vi "TruncU64.vi"(5 "Decimal places":i8, 6 "Number":u64) -> (2 "Truncated number":u64)   [LabVIEW 2017, in "GPNumeric.lvlib"]
doc: "Truncates <B>Number</B> to a number of <B>Decimal places</B>.\n\nSet <B>Decimal places</B> to a negative number to truncate to nearest 10, nearest 100 and so on. E.g. to truncate 782 to the nearest hundred, you set <B>Decimal places</B> to -2 and the <B>Truncated number</B> will be 700.\n\nThis VI is inlined.\n\nSteen Schmidt\nGPower\n16/5 2014"
uses:
  GPNumeric.lvlib
panel:
  # "Copyright © 2014\nGPower\nSee enclosed license file for terms and conditions"
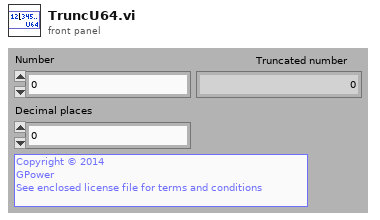
[diagram p1: front panel]
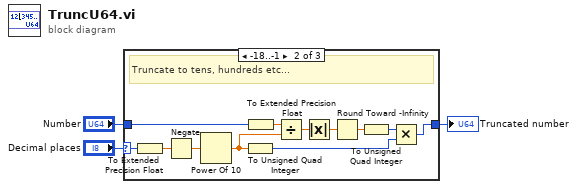
[diagram p0: block diagram]
diagram:
  n1 = case shown="-18..-1" "Decimal places" {
    selector: "Decimal places" -> [_ w12 _]
    tunnel: [_ w9 w16] -> w3
    tunnel: "Number" -> [_ w10 w16]
    frame ..-19 {
      # "Truncate above max value; Return zero."
    }
    frame -18..-1 {
      # "Truncate to tens, hundreds etc..."
      n2 = To Extended Precision Float(1:w12) -> (0:w11:ext)
      n3 = Negate(x=w11) -> (-x=w15:ext)
      n4 = Power Of 10(x=w15) -> (10^x=w8:ext)
      n5 = To Unsigned Quad Integer(1:w8) -> (0:w14:u64)
      n6 = To Extended Precision Float(1:w10) -> (0:w6:ext)
      n7 = Divide(x=w6, y=w8) -> (x/y=w5:ext)
      n8 = Absolute Value(x=w5) -> (abs(x)=w7:ext)
      n9 = Round Toward -Infinity(1:w7) -> (0:w4:ext)
      n10 = To Unsigned Quad Integer(1:w4) -> (0:w13:u64)
      n11 = Multiply(x=w13, y=w14) -> (x*y=w9:u64)
    }
    frame 0.. {
      # "Truncate to n decimal places; return integer unchanged."
    }
  }
  "Truncated number" <- w3
